vi "2012 Target Simulator.vi"() -> ()   [LabVIEW 2011]
uses:
  <vilib>/Rock Robotics/WPI/Camera/WPI_CameraImageSize.ctl
  <vilib>/addons/control/pid/NI_PID_pid.lvlib
panel:
  in  "reinitialize? (F)":bool
  out "Target Angle":dbl
  out "Waveform Chart":dbl(graph)
  in  "Gyro Angle (deg)":dbl(knob)=3.7731857266145283 scale=-45.0..45.0
  out "Rotation":dbl=-0.26122391808015843
  in  "saturation Gyro":dbl=0.7
  in  "PID gains Gyro":T1={"proportional gain (Kc)"=0.03, "integral time (Ti, min)"=0.01, "derivative time (Td, min)"=0.002} {"derivative time (Td, min)" format="%#.7g"; "integral time (Ti, min)" format="%#.6g"; "proportional gain (Kc)" format="%#.6g"}
  in  "# of Targets":dbl=1.0 min=1.0 max=4.0 step=1.0
  in  "stop":bool
  in  "Decimate by":cluster{"H":i32, "V":i32}={"H"=1, "V"=1}
  in  "Camera Type":enum16{"206", "1011"}(ring)
  in  "Image Size":T2=enum."320x240"
  in  "Score Limits":T3={"Rect Coverage"=76.0, "Aspect Ratio"=70.0, "X Edge Strength"=40.0, "Y Edge Strength"=60.0}
  out "Top Goal":T4
  out "Top Goal":T5
  out "Min Top":dbl
  out "Target Info":T6(array[cluster])
  out "Distance":dbl format="%#_4g"
  out "x+y":dbl
  out "x*y":dbl
  out "Position.X":dbl
  out "Index":i32
  in  "cluster":T7
  in  "4 Targets":T8(array[cluster])=[{{"Left"=135.0, "Top"=40.0, "Right"=185.0, "Bottom"=77.5}, []}, {{"Left"=94.6, "Top"=117.1, "Right"=144.6, "Bottom"=154.6}, []}, {{"Left"=175.4, "Top"=117.1, "Right"=225.4, "Bottom"=154.6}, []}, {{"Left"=135.0, "Top"=185.8, "Right"=185.0, "Bottom"=223.3}, []}]
  in  "1 Target":T8(array[cluster])
  in  "2 Targets":T8(array[cluster])
  in  "3 targets":T8(array[cluster])
  # "Outputs"
  # "Simultated Targets"
  # "Bottom"
  # "Top"
  # "Right"
  # "Left"
  # "Rotate to Target Simulator"
  # "Vision Inputs"
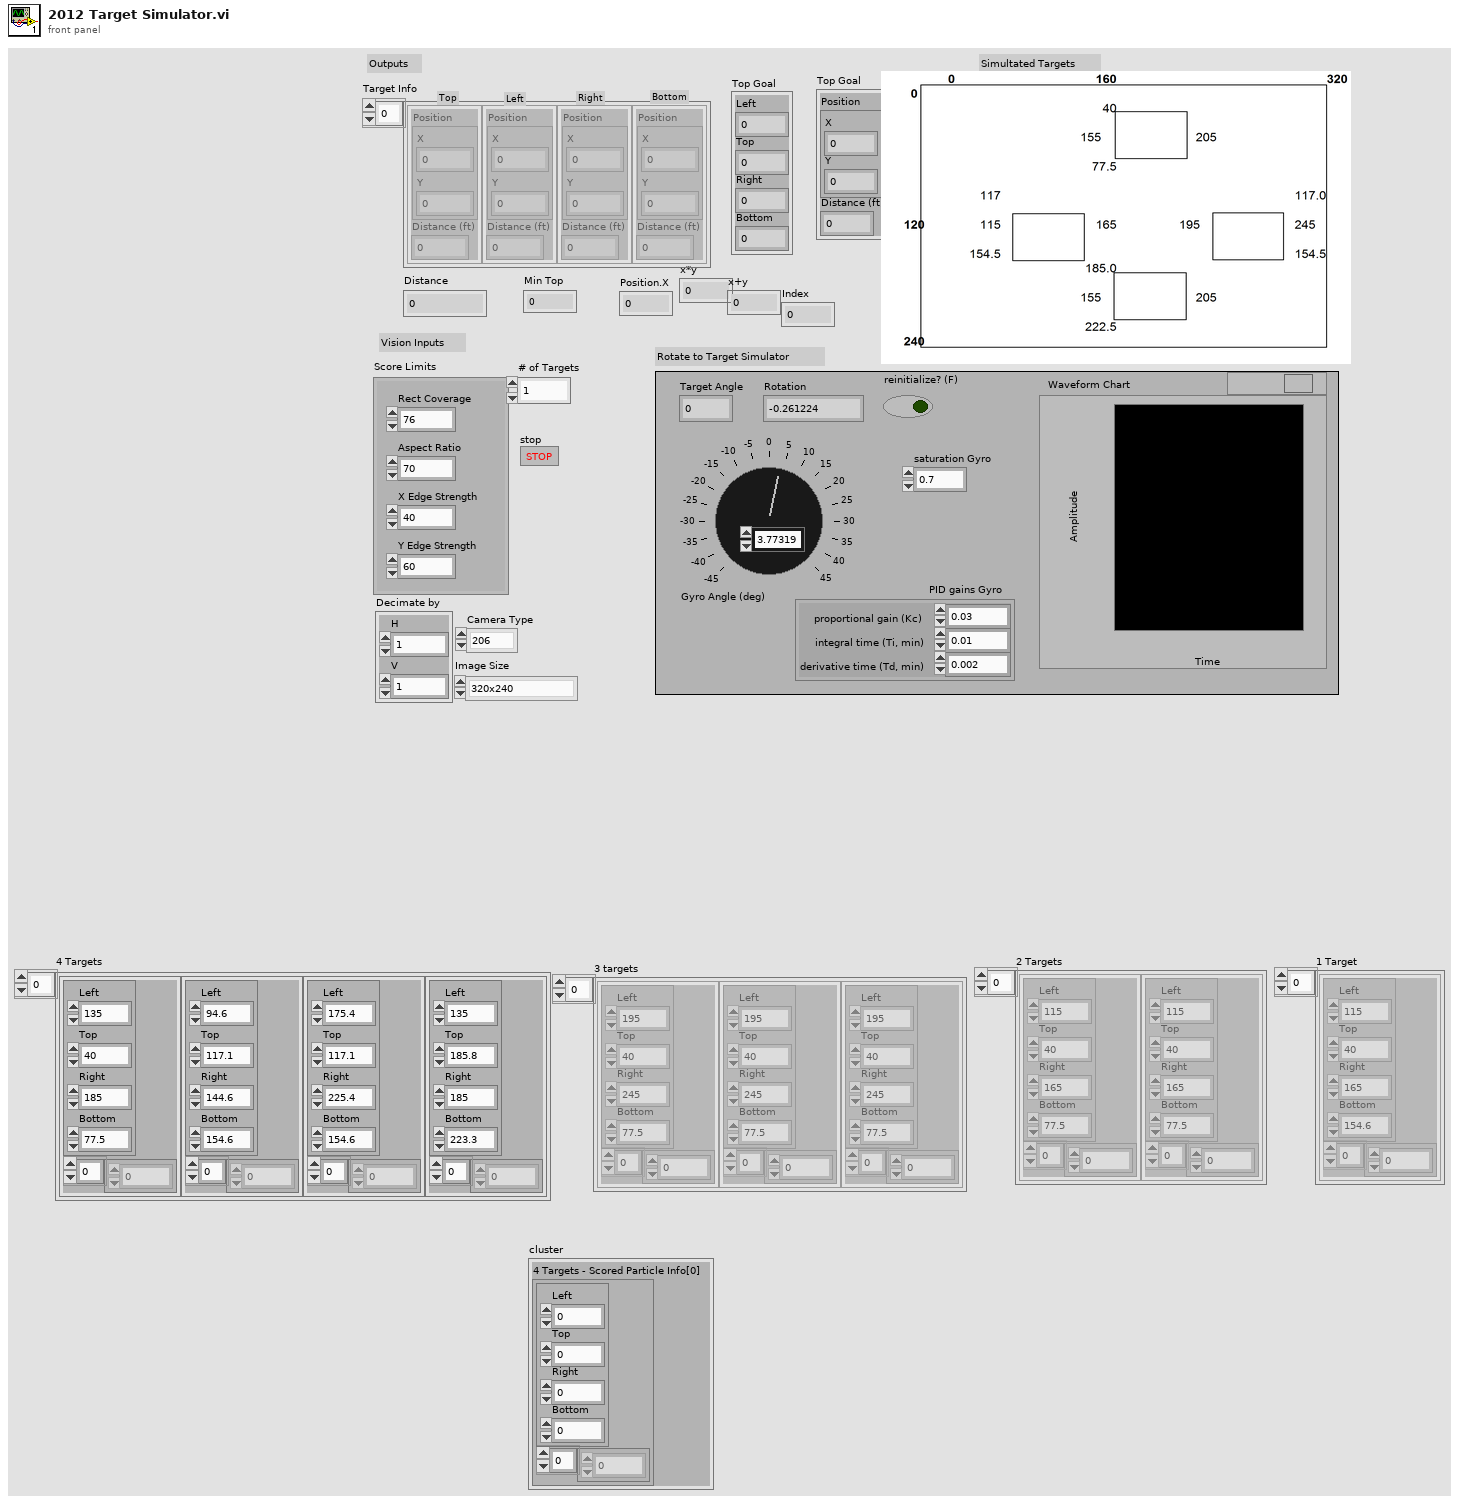
[diagram p1: front panel]
types:
  T1 = cluster{"proportional gain (Kc)":dbl, "integral time (Ti, min)":dbl, "derivative time (Td, min)":dbl}
  T2 = typedef "WPI_CameraImageSize.ctl" = enum16{"640x480", "320x240", "160x120"}
  T3 = cluster{"Rect Coverage":dbl, "Aspect Ratio":dbl, "X Edge Strength":dbl, "Y Edge Strength":dbl}
  T4 = cluster{"Position":cluster{"X":dbl, "Y":dbl}, "Distance (ft)":dbl}
  T5 = cluster{"Left":dbl, "Top":dbl, "Right":dbl, "Bottom":dbl}
  T6 = cluster{"Position":cluster{"X":dbl, "Y":dbl}, "Distance (ft)":dbl}[]
  T7 = cluster{"4 Targets - Scored Particle Info[0]":cluster{cluster{"Left":dbl, "Top":dbl, "Right":dbl, "Bottom":dbl}, dbl[]}}
  T8 = cluster{cluster{"Left":dbl, "Top":dbl, "Right":dbl, "Bottom":dbl}, dbl[]}[]
  T9 = cluster{"Target Center (-1 to 1)":cluster{"X":dbl, "Y":dbl}, "Distance (ft)":dbl}
  T10 = cluster{"Target Center (-1 to 1)":cluster{"X":dbl, "Y":dbl}, "Distance (ft)":dbl}[]
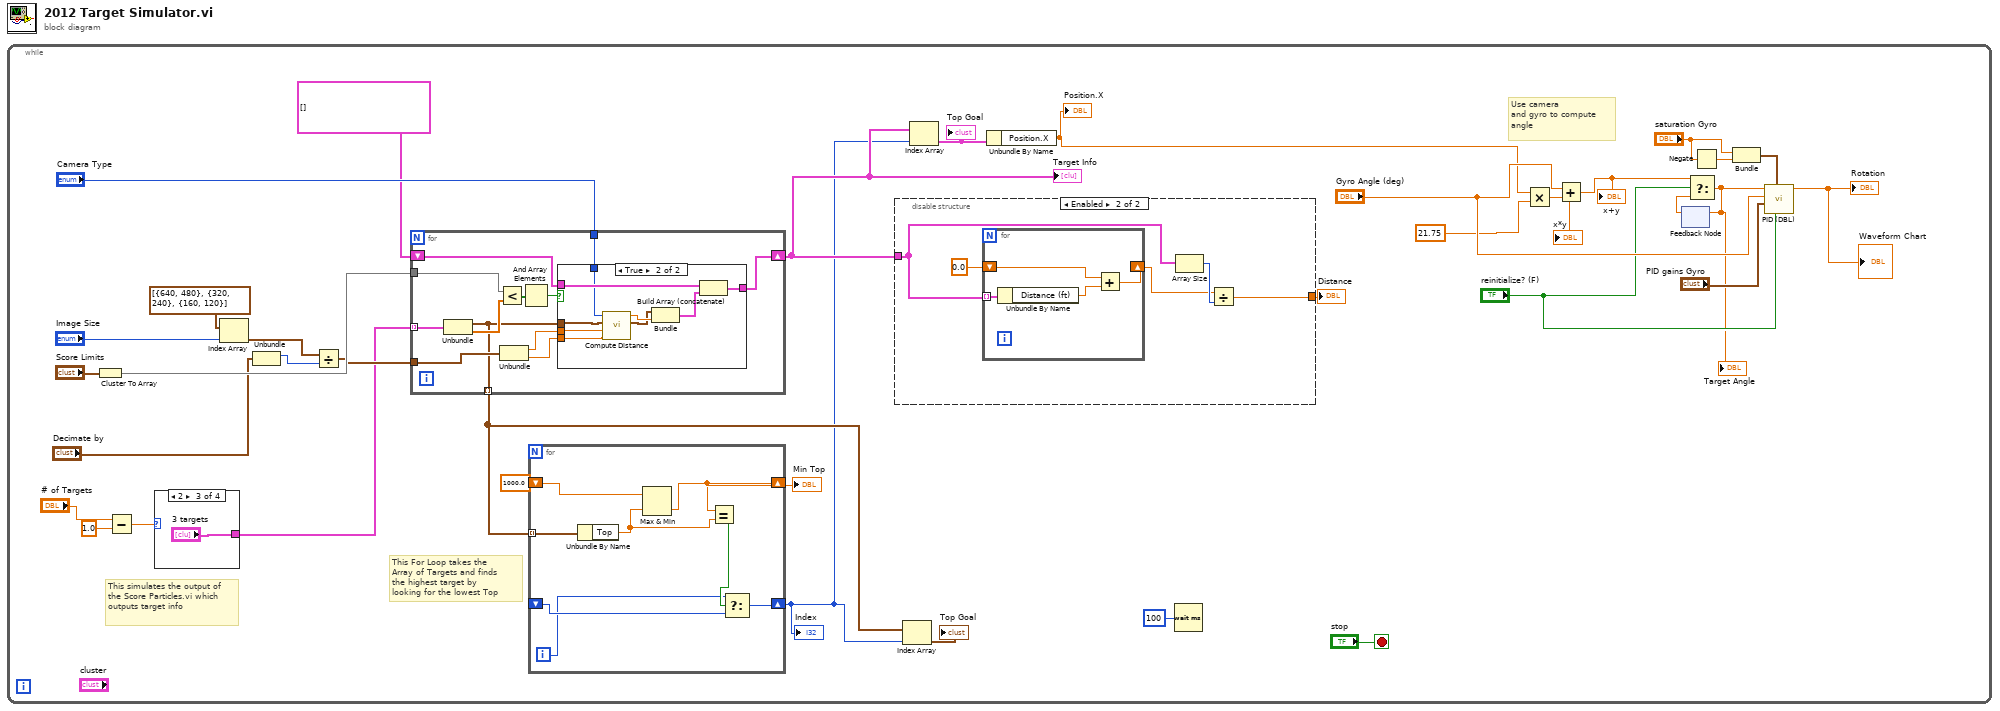
[diagram p0: block diagram]
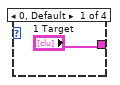
[diagram p2: hidden frame]
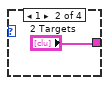
[diagram p3: hidden frame]
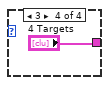
[diagram p4: hidden frame]
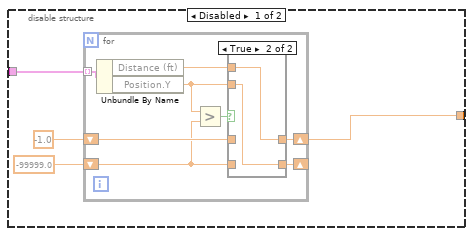
[diagram p5: hidden frame]
diagram:
  n1 = while {
    stop <- "stop" stop-if-true
    # "This For Loop takes the Array of Targets and finds the highest target by looking for the lowest Top"
    # "This simulates the output of the Score Particles.vi which outputs target info"
    # "Use camera\nand gyro to compute\nangle"
    n2 = Cluster To Array(cluster="Score Limits") -> (array=w33:dbl[])
    n3 = Subtract(x="# of Targets", y=1.0) -> (x-y=w22:dbl)
    n4 = case shown="2" w22 {
      tunnel: ["1 Target" "2 Targets" "3 targets" "4 Targets"] -> w23
      frame 0, Default {
      }
      frame 1 {
      }
      frame 2 {
      }
      frame 3 {
      }
    }
    n5 = Index Array(array=cluster{i32, i32}[] [{640, 480}, {320, 240}, {160, 120}], index="Image Size") -> (element=w32:cluster{i32, i32})
    n6 = Unbundle("Decimate by") -> ("H"=w25:i32)  [unwired: 1 out]
    n7 = Divide(x=w32, y=w25) -> (x/y=w31:cluster{dbl, dbl})
    n8 = for {
      tunnel: w33 -> [w85]
      tunnel: w31 -> [w82]
      tunnel: "Camera Type" -> [w79]
      shift-right: [w77] -> w16
      shift-left: T6 [] -> [w78]
      tunnel: w23 -> [w76] mode=indexing
      tunnel: [w75] -> w18 mode=indexing
      n9 = Unbundle(w76) -> (w75:T5, w86:dbl[])
      n10 = Less?(x=w85, y=w86) -> (x < y?=w84:bool[])
      n11 = Unbundle(w82) -> (w81:dbl, w80:dbl)
      n12 = And Array Elements(Boolean array=w84) -> (logical AND=w83:bool)
      n13 = case shown="True" w83 {
        tunnel: w81 -> [_ w92]
        tunnel: w80 -> [_ w93]
        tunnel: w75 -> [_ w91]
        tunnel: w79 -> [_ w90]
        tunnel: w78 -> [w87 w96]
        tunnel: [w87 w95] -> w77
        frame False {
        }
        frame True {
          n14 = call "Compute Distance.vi"("Y Image Resolution"=w93, "X Image Resolution"=w92, "Bounding Box"=w91, "Camera Type"=w90) -> ("Target Center (-1 to 1)"=w88:cluster{"X":dbl, "Y":dbl}, "Distance (ft)"=w94:dbl)  [unwired: 6 in]
          n15 = Bundle("Target Center (-1 to 1)"=w88, "Distance (ft)"=w94) -> (w89:T9)  [unwired: 1 in]
          n16 = Build Array (concatenate)(w96, w89) -> (w95:T10)
        }
      }
    }
    "Target Info" <- w16
    n17 = for {
      shift-right: [w47] -> w19
      shift-left: 1000.0 -> [w49]
      tunnel: w18 -> [w48] mode=indexing
      shift-right: [w44] -> w15
      shift-left: _ -> [w43]
      i -> [w42]
      n18 = Unbundle By Name(w48) -> ("Top"=w45:dbl)
      n19 = Max & Min(x=w49, y=w45) -> (min(x,y)=w47:dbl)  [unwired: 1 out]
      n20 = Equal?(x=w47, y=w45) -> (x = y?=w46:bool)
      n21 = Select(t=w42, s=w46, f=w43) -> (s? t:f=w44:i32)
    }
    "Min Top" <- w19
    "Index" <- w15
    n22 = disable-structure shown="Enabled" {
      disable-tunnel: w16 -> [w51 w67]
      disable-tunnel: [w50 w66] -> w30
      frame Disabled {
        n23 = for {
          tunnel: w51 -> [w61] mode=indexing
          shift-right: [w57] -> w50
          shift-left: -1.0 ("y") -> [w58]
          shift-right: [w59] -> _
          shift-left: -99999.0 ("y") -> [w56]
          n24 = Unbundle By Name(w61) -> ("Distance (ft)"=w55:dbl, "Position.Y"=w54:dbl)
          n25 = Greater?(x=w54, y=w56) -> (0:w60:bool)
          n26 = case shown="True" w60 {
            tunnel: w56 -> [w63 _]
            tunnel: [w63 w65] -> w59
            tunnel: [w62 w64] -> w57
            tunnel: w58 -> [w62 _]
            tunnel: w55 -> [_ w64]
            tunnel: w54 -> [_ w65]
            frame False {
            }
            frame True {
            }
          }
        }
      }
      frame Enabled {
        n27 = for {
          tunnel: w67 -> [w74] mode=indexing
          shift-right: [w72] -> w68
          shift-left: 0.0 -> [w71]
          n28 = Unbundle By Name(w74) -> ("Distance (ft)"=w73:dbl)
          n29 = Add(x=w71, y=w73) -> (x+y=w72:dbl)
        }
        n30 = Array Size(array=w67) -> (size(s)=w69:i32)
        n31 = Divide(x=w68, y=w69) -> (x/y=w66:dbl)
      }
    }
    "Distance" <- w30
    n32 = Index Array(array=w18, index=w15) -> (element=→"Top Goal":T5)
    n33 = Index Array(array=w16, index=w15) -> (element=w14:T4)
    "Top Goal" <- w14
    n34 = Unbundle By Name(w14) -> ("Position.X"=w7:dbl)
    "Position.X" <- w7
    n35 = Wait (ms)(milliseconds to wait=u32 100) -> ()  [unwired: 1 out]
    n36 = Multiply(x=w7, y=sgl 21.75 ("deg full screen 2")) -> (x*y=w5:dbl)
    "x*y" <- w5
    n37 = Add(x="Gyro Angle (deg)", y=w5) -> (x+y=w3:dbl)
    "x+y" <- w3
    n38 = feedback #1() -> (w4:dbl)  [unwired: 1 out]
    n39 = Select(t=w3, s="reinitialize? (F)", f=w4) -> (s? t:f=w1:dbl)
    "Target Angle" <- w1
    n40 = feedback-in #1(w1) -> ()
    n41 = Negate(x="saturation Gyro") -> (-x=w12:dbl)
    n42 = Bundle("saturation Gyro"="saturation Gyro", w12) -> (w9:cluster{"saturation Gyro":dbl, dbl})  [unwired: 1 out]
    n43 = call <vilib>:"PID (DBL).vi"("reinitialize? (F)"="reinitialize? (F)", "output range"=w9, "PID gains"="PID gains Gyro", "process variable"="Gyro Angle (deg)", "setpoint"=w1) -> ("output"=→"Rotation" →"Waveform Chart":dbl)  [unwired: 1 in, 5 out]
  }
